vi "Runtime Menue Text aendern.vi"(8 "Fehler (Eingang, kein Fehler)":errorcluster, 11 "Menüreferenz":refnum<k9>) -> (0 "Fehler (Ausgang)":errorcluster)   [LabVIEW 2020, in "Sprachverwaltung.lvlib"]
uses:
  Sprachverwaltung.lvlib
  FGV Aktion Tabelle zerlegen.ctl
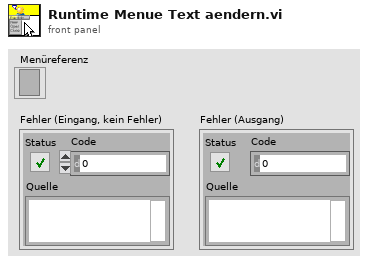
[diagram p1: front panel]
types:
  T1 = typedef "Sprachverwaltung.lvlib/FGV Aktion Tabelle zerlegen.ctl" = enum16{"laden", "vereinzeln", "speichern"}
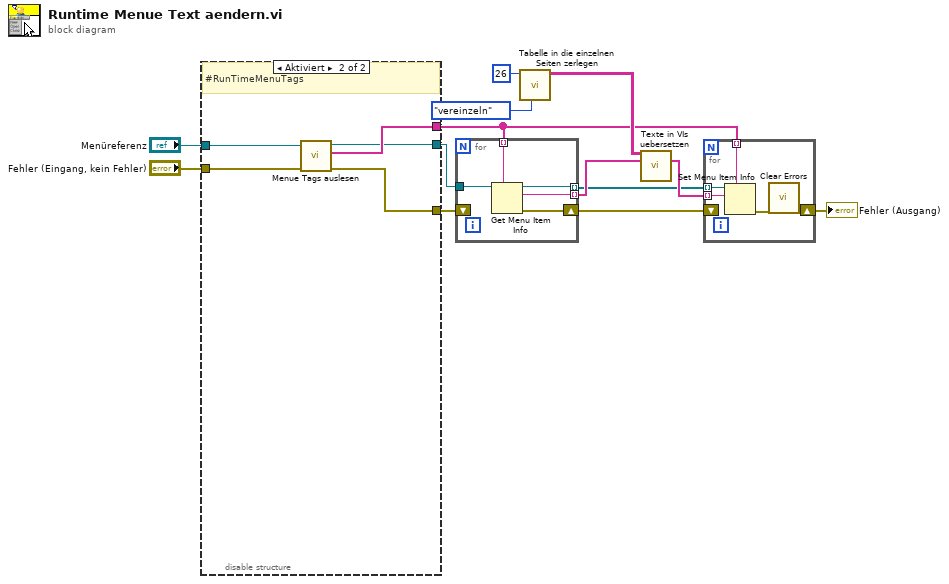
[diagram p0: block diagram]
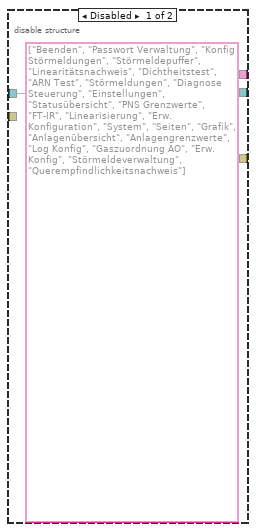
[diagram p2: hidden frame]
diagram:
  n1 = disable-structure shown="Aktiviert" {
    disable-tunnel: [string[] ["Beenden", "Passwort Verwaltung", "Konfig Störmeldungen", "Störmeldepuffer", "Linearitätsnachweis", "Dichtheitstest", "ARN Test", "Störmeldungen", "Diagnose Steuerung", "Einstellungen", "Statusübersicht", "PNS Grenzwerte", "FT-IR", "Linearisierung", "Erw. Konfiguration", "System", "Seiten", "Grafik", "Anlagenübersicht", "Anlagengrenzwerte", "Log Konfig", "Gaszuordnung AO", "Erw. Konfig", "Störmeldeverwaltung", "Querempfindlichkeitsnachweis"] w18] -> w8
    disable-tunnel: "Menüreferenz" -> [w14 w20]
    disable-tunnel: "Fehler (Eingang, kein Fehler)" -> [_ w19]
    disable-tunnel: [w14 w17] -> w4
    disable-tunnel: [_ w16] -> w3
    frame Disabled {
    }
    frame Enabled {
      # "#RunTimeMenuTags"
      n2 = call "Menue Tags auslesen.vi"("error in (no error)"=w19, "Menü Referenz"=w20) -> ("error out"=w16:errorcluster, "Menu Tags"=w18:string[], "Menü Referenz out"=w17:refnum<k9>)  [unwired: 7 in]
    }
  }
  n3 = for {
    tunnel: w4 -> [w25]
    tunnel: [w24] -> w9 mode=indexing
    tunnel: w8 -> [w23] mode=indexing
    tunnel: [w22] -> w11 mode=indexing
    shift-right: [w21] -> w2
    shift-left: w3 -> [_]
    n4 = Get Menu Item Info(7:w23, 11:w25) -> (0:w21:errorcluster, 2:w22:string, 3:w24:refnum<k9>)  [unwired: 1 in, 4 out]
  }
  n5 = call "Tabelle in die einzelnen Seiten zerlegen.vi"("Aktion"=FGV_Aktion_Tabelle_zerlegen."vereinzeln", "Index (Seite)"=26) -> ("Sprachliste"=w12:string[][])  [unwired: 7 in, 2 out]
  n6 = call "Texte in VIs uebersetzen.vi"("Sprachliste"=w12, "String-Array zum Übersetzen"=w11) -> ("String-Array zum Übersetzen"=w10:string[])  [unwired: 9 in, 4 out]
  n7 = for {
    tunnel: w9 -> [w30] mode=indexing
    tunnel: w8 -> [w29] mode=indexing
    tunnel: w10 -> [w28] mode=indexing
    shift-right: [w26] -> w1
    shift-left: w2 -> [_]
    n8 = Set Menu Item Info(7:w29, 10:w28, 11:w30) -> (0:w27:errorcluster)  [unwired: 4 in, 1 out]
    n9 = call <vilib>:"Clear Errors.vi"("error in (no error)"=w27) -> ("error out"=w26:errorcluster)  [unwired: 5 in, 1 out]
  }
  "Fehler (Ausgang)" <- w1
